vi "AKD Initialise.vi"(0 "Connection Settings":T1, 5 "Stop drive":bool=TRUE, 11 "error in":errorcluster) -> (4 "connection ID":refnum<k5>, 15 "error out":errorcluster)   [LabVIEW 2024]
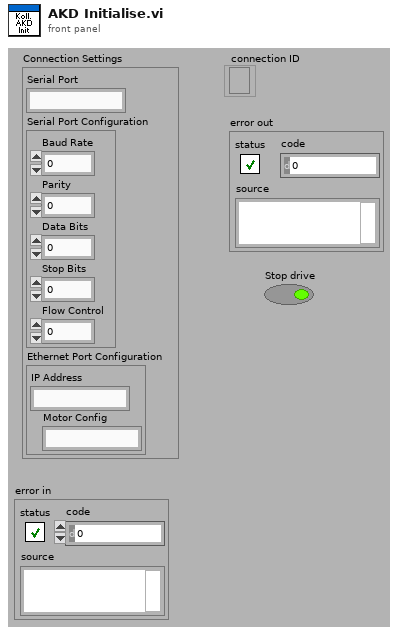
[diagram p1: front panel]
types:
  T1 = cluster{"Serial Port":string, "Serial Port Configuration":cluster{"Baud Rate":u32, "Parity":u16, "Data Bits":u16, "Stop Bits":u16, "Flow Control":u16}, "Ethernet Port Configuration":cluster{"IP Address":string, "Motor Config":string}}
  T2 = cluster{"IP Address":string, "Motor Config":string}
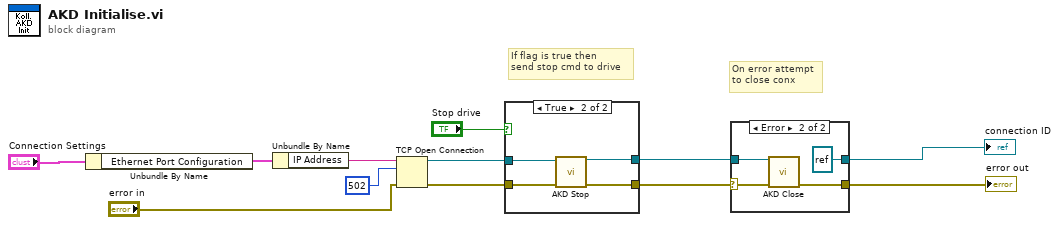
[diagram p0: block diagram]
diagram:
  # "On error attempt\nto close conx"
  # "If flag is true then\nsend stop cmd to drive"
  n1 = Unbundle By Name("Connection Settings") -> ("Ethernet Port Configuration"=w8:T2)
  n2 = Unbundle By Name(w8) -> ("IP Address"=w10:string)
  n3 = TCP Open Connection(address=w10, remote port or service name=u16 502, error in (no error)="error in") -> (connection ID=w2:refnum<k5>, error out=w5:errorcluster)  [unwired: 2 in]
  n4 = case shown="True" "Stop drive" {
    tunnel: w5 -> [w14 w18]
    tunnel: [w14 w17] -> w4
    tunnel: [w13 w16] -> w3
    tunnel: w2 -> [w13 w15]
    frame False {
    }
    frame True {
      n5 = call "AKD Stop.vi"("connection ID"=w15, "error in"=w18) -> ("TCP Refnum"=w16:refnum<k5>, "error out"=w17:errorcluster)  [unwired: 12 in]
    }
  }
  n6 = case shown="Error" w4 {
    selector: w4 -> [w19 w23]
    tunnel: w3 -> [w20 w24]
    tunnel: [w19 w22] -> w7
    tunnel: [w20 refnum<k5> refnum ("TCP Refnum")] -> w6
    frame No Error {
    }
    frame Error {
      n7 = call "AKD Close.vi"("connection ID"=w24, "error in"=w23) -> ("error out"=w22:errorcluster)  [unwired: 13 in]
    }
  }
  "error out" <- w7
  "connection ID" <- w6
